vi "Set Tree Symbols.vi"(8 "error in":errorcluster, 10 "Tag":string, 11 "CtlRef":refnum<vi>) -> (0 "error out":errorcluster)   [LabVIEW 2015, in "J1939 Addon System Explorer.lvlib"]
uses:
  J1939 Addon System Explorer.lvlib
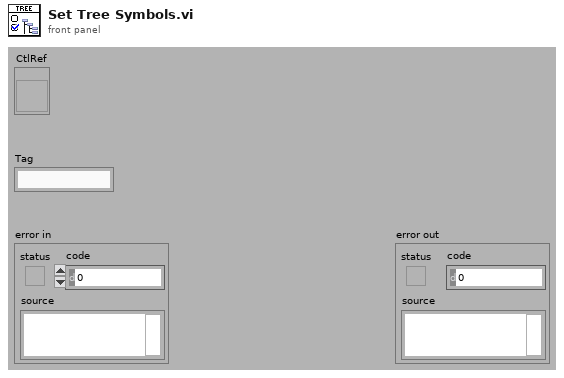
[diagram p1: front panel]
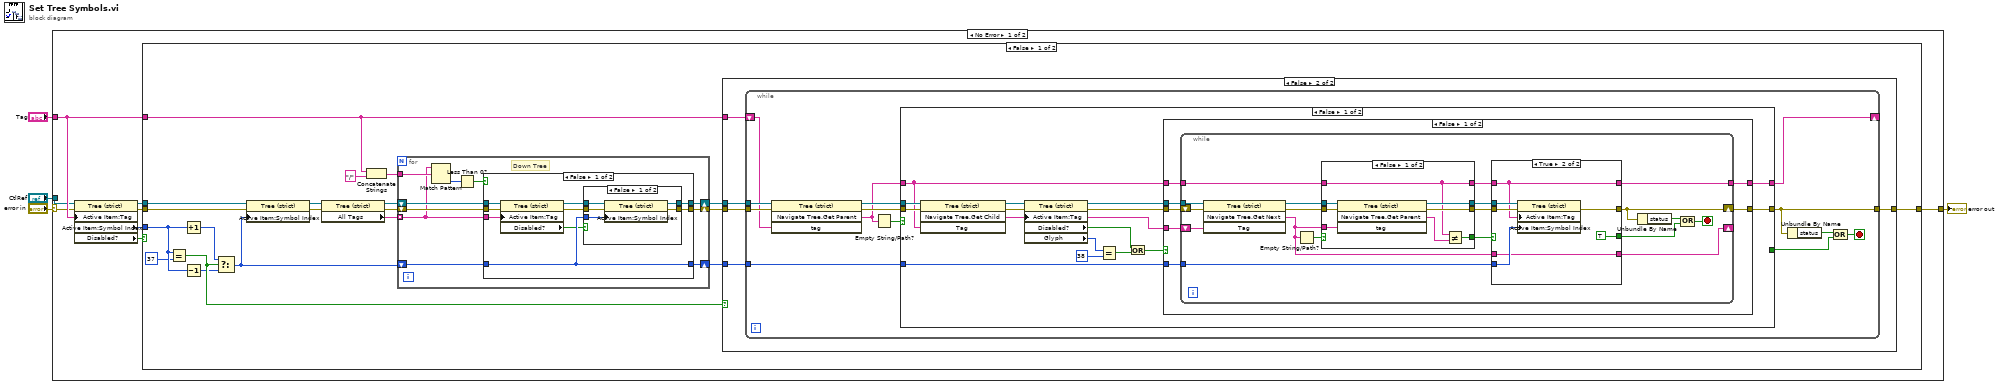
[diagram p0: block diagram]
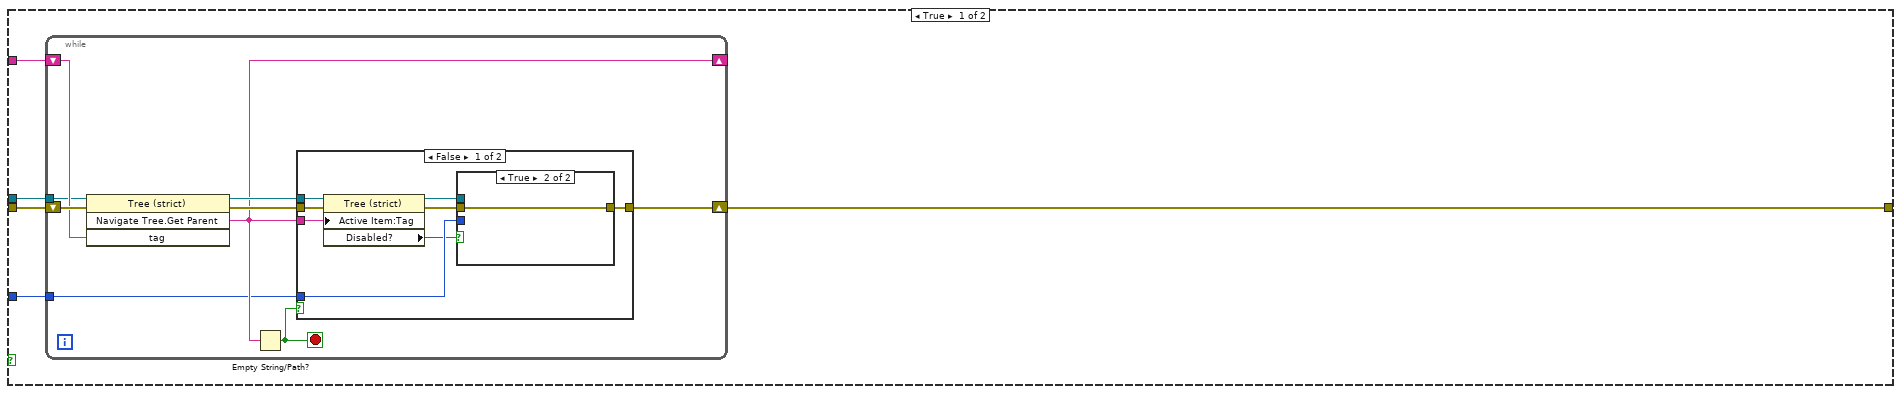
[diagram p2: hidden frame]
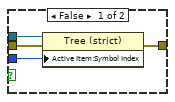
[diagram p3: hidden frame]
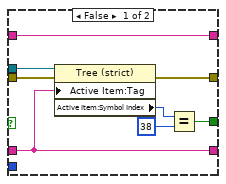
[diagram p6: hidden frame]
diagram:
  n1 = case shown="No Error" "error in" {
    selector: "error in" -> [w6 w183]
    tunnel: [w12 w183] -> w4
    tunnel: "Tag" -> [w11 _]
    tunnel: "CtlRef" -> [w10 _]
    frame No Error {
      n2 = property class="Tree (strict)"(reference=w10, error in=w6, "Active Item:Tag"=w11) -> (reference out=w8:refnum<vi>, error out=w9:errorcluster, "Active Item:Symbol Index"=w7:i32, "Disabled?"=w5:bool)
      n3 = case shown="False" w5 {
        tunnel: [w31 w182] -> w12
        tunnel: w11 -> [w29 _]
        tunnel: w9 -> [w18 w182]
        tunnel: w8 -> [w17 _]
        tunnel: w7 -> [w15 _]
        frame False {
          n4 = Equal?(x=w15, y=37 ("Active Item:Symbol Index")) -> (x = y?=w26:bool)
          n5 = Increment(x=w15) -> (x+1=w14:i32)
          n6 = Decrement(x=w15) -> (x-1=w16:i32)
          n7 = Select(t=w14, s=w26, f=w16) -> (s? t:f=w27:i32)
          n8 = property class="Tree (strict)"(reference=w17, error in=w18, "Active Item:Symbol Index"=w27) -> (reference out=w19:refnum<vi>, error out=w20:errorcluster)
          n9 = property class="Tree (strict)"(reference=w19, error in=w20) -> (reference out=w22:refnum<vi>, error out=w21:errorcluster, "All Tags"=w25:string[])
          n10 = Concatenate Strings(w29, "/" ("string")) -> (w24:string)
          n11 = for {
            tunnel: w24 -> [w162]
            tunnel: w25 -> [w155] mode=indexing
            shift-right: [w158] -> w28
            shift-left: w21 -> [w157]
            shift-right: [w154] -> w30
            shift-left: w22 -> [w156]
            shift-right: [w153] -> w32
            shift-left: w27 -> [w159]
            # "Down Tree"
            n12 = Match Pattern(string=w155, regular expression=w162) -> (offset past match=w161:i32)  [unwired: 1 in, 3 out]
            n13 = Less Than 0?(x=w161) -> (x < 0?=w160:bool)
            n14 = case shown="False" w160 {
              tunnel: w157 -> [w170 w181]
              tunnel: w156 -> [w171 w180]
              tunnel: w155 -> [w169 _]
              tunnel: w159 -> [w164 w179]
              tunnel: [w165 w181] -> w158
              tunnel: [w166 w180] -> w154
              tunnel: [w164 w179] -> w153
              frame False {
                n15 = property class="Tree (strict)"(reference=w171, error in=w170, "Active Item:Tag"=w169) -> (reference out=w167:refnum<vi>, error out=w168:errorcluster, "Disabled?"=w163:bool)
                n16 = case shown="False" w163 {
                  tunnel: w168 -> [w176 w177]
                  tunnel: w167 -> [w175 w178]
                  tunnel: [w174 w178] -> w166
                  tunnel: [w173 w177] -> w165
                  tunnel: w164 -> [w172 _]
                  frame False {
                    n17 = property class="Tree (strict)"(reference=w175, error in=w176, "Active Item:Symbol Index"=w172) -> (reference out=w174:refnum<vi>, error out=w173:errorcluster)
                  }
                  frame True {
                  }
                }
              }
              frame True {
              }
            }
          }
          n18 = case shown="False" w26 {
            tunnel: w28 -> [w37 w64]
            tunnel: w29 -> [w36 w62]
            tunnel: w30 -> [w35 w63]
            tunnel: [w34 w65] -> w31
            tunnel: w32 -> [w33 w61]
            frame True {
              n19 = while {
                tunnel: w35 -> [w44]
                shift-right: [w39] -> w34
                shift-left: w37 -> [w46]
                shift-right: [w41] -> _
                shift-left: w36 -> [w45]
                tunnel: w33 -> [w40]
                stop <- w38 stop-if-true
                n20 = invoke on="Invoke Node" class="Tree (strict)" method="Navigate Tree.Get Parent"(reference=w44, error in=w46, "tag"=w45) -> (reference out=w43:refnum<vi>, error out=w42:errorcluster, "Navigate Tree:Get Parent"=w41:string)  [unwired: 1 in, 1 out]
                n21 = Empty String/Path?(string/path=w41) -> (empty?=w38:bool)
                n22 = case shown="False" w38 {
                  tunnel: w42 -> [w53 w60]
                  tunnel: w43 -> [w54 _]
                  tunnel: w41 -> [w52 _]
                  tunnel: w40 -> [w48 _]
                  tunnel: [w49 w60] -> w39
                  frame False {
                    n23 = property class="Tree (strict)"(reference=w54, error in=w53, "Active Item:Tag"=w52) -> (reference out=w50:refnum<vi>, error out=w51:errorcluster, "Disabled?"=w47:bool)
                    n24 = case shown="True" w47 {
                      tunnel: w51 -> [w58 w59]
                      tunnel: w50 -> [w57 _]
                      tunnel: [w56 w59] -> w49
                      tunnel: w48 -> [w55 _]
                      frame False {
                        n25 = property class="Tree (strict)"(reference=w57, error in=w58, "Active Item:Symbol Index"=w55) -> (error out=w56:errorcluster)  [unwired: 1 out]
                      }
                      frame True {
                      }
                    }
                  }
                  frame True {
                  }
                }
              }
            }
            frame False {
              n26 = while {
                tunnel: [w69] -> w65
                tunnel: w64 -> [w78]
                tunnel: w63 -> [w77]
                shift-right: [w72] -> _
                shift-left: w62 -> [w71]
                tunnel: w61 -> [w70]
                stop <- w67 stop-if-true
                n27 = invoke on="Invoke Node" class="Tree (strict)" method="Navigate Tree.Get Parent"(reference=w77, error in=w78, "tag"=w71) -> (reference out=w75:refnum<vi>, error out=w76:errorcluster, "Navigate Tree:Get Parent"=w74:string)  [unwired: 1 in, 1 out]
                n28 = Empty String/Path?(string/path=w74) -> (empty?=w73:bool)
                n29 = case shown="False" w73 {
                  selector: w73 -> [_ w150]
                  tunnel: w70 -> [w94 _]
                  tunnel: [w93 w152] -> w69
                  tunnel: w76 -> [w92 w152]
                  tunnel: w75 -> [w91 _]
                  tunnel: w74 -> [w86 w151]
                  tunnel: [w84 w151] -> w72
                  tunnel: [_ w150] -> w66
                  frame False {
                    n30 = invoke on="Invoke Node" class="Tree (strict)" method="Navigate Tree.Get Child"(reference=w91, error in=w92, "Tag"=w86) -> (reference out=w90:refnum<vi>, error out=w88:errorcluster, "Navigate Tree:Get Child"=w79:string)  [unwired: 1 in, 1 out]
                    n31 = property class="Tree (strict)"(reference=w90, error in=w88, "Active Item:Tag"=w79) -> (reference out=w89:refnum<vi>, error out=w87:errorcluster, "Disabled?"=w82:bool, "Glyph"=w83:i32)
                    n32 = Equal?(x=w83, y=38 ("Active Item:Symbol Index")) -> (x = y?=w81:bool)
                    n33 = Or(x=w82, y=w81) -> (x .or. y?=w80:bool)
                    n34 = case shown="False" w80 {
                      tunnel: w94 -> [w101 _]
                      tunnel: [w100 w149] -> w93
                      tunnel: w89 -> [w99 _]
                      tunnel: w87 -> [w98 w149]
                      tunnel: w79 -> [w97 _]
                      tunnel: w86 -> [w96 w148]
                      tunnel: [w95 w148] -> w84
                      frame False {
                        n35 = while {
                          tunnel: w101 -> [w120]
                          tunnel: w99 -> [w117]
                          shift-right: [w107] -> w100
                          shift-left: w98 -> [w119]
                          shift-right: [w102] -> _
                          shift-left: w97 -> [w118]
                          tunnel: w96 -> [w108]
                          tunnel: [w103] -> w95
                          stop <- w105 stop-if-true
                          n36 = invoke on="Invoke Node" class="Tree (strict)" method="Navigate Tree.Get Next"(reference=w117, error in=w119, "Tag"=w118) -> (reference out=w116:refnum<vi>, error out=w114:errorcluster, "Navigate Tree:Get Next Item"=w109:string)  [unwired: 1 in, 1 out]
                          n37 = Empty String/Path?(string/path=w109) -> (empty?=w111:bool)
                          n38 = case shown="False" w111 {
                            selector: w111 -> [_ w132]
                            tunnel: w116 -> [w128 w130]
                            tunnel: [w127 w130] -> w115
                            tunnel: w114 -> [w126 w131]
                            tunnel: [w125 w131] -> w113
                            tunnel: [w123 w132] -> w112
                            tunnel: w108 -> [w121 w129]
                            tunnel: w109 -> [w122 _]
                            tunnel: [w121 w129] -> w110
                            frame False {
                              n39 = invoke on="Invoke Node" class="Tree (strict)" method="Navigate Tree.Get Parent"(reference=w128, error in=w126, "tag"=w122) -> (reference out=w127:refnum<vi>, error out=w125:errorcluster, "Navigate Tree:Get Parent"=w124:string)  [unwired: 1 in, 1 out]
                              n40 = Not Equal?(x=w121, y=w124) -> (x != y?=w123:bool)
                            }
                            frame True {
                            }
                          }
                          n41 = case shown="True" w112 {
                            tunnel: w120 -> [_ w143]
                            tunnel: w113 -> [w140 w145]
                            tunnel: [w135 w146] -> w107
                            tunnel: w115 -> [w139 w144]
                            tunnel: w109 -> [w133 w141]
                            tunnel: [w136 TRUE] -> w104
                            tunnel: w110 -> [w134 w142]
                            tunnel: [w134 w142] -> w103
                            tunnel: [w133 w141] -> w102
                            frame False {
                              n42 = property class="Tree (strict)"(reference=w139, error in=w140, "Active Item:Tag"=w133) -> (error out=w135:errorcluster, "Active Item:Symbol Index"=w137:i32)  [unwired: 1 out]
                              n43 = Equal?(x=w137, y=38 ("Active Item:Symbol Index")) -> (x = y?=w136:bool)
                            }
                            frame True {
                              n44 = property class="Tree (strict)"(reference=w144, error in=w145, "Active Item:Tag"=w142, "Active Item:Symbol Index"=w143) -> (error out=w146:errorcluster)  [unwired: 1 out]
                            }
                          }
                          n45 = Unbundle By Name(w107) -> ("status"=w106:bool)
                          n46 = Compound Arithmetic op=OR(w106, w104) -> (w105:bool)
                        }
                      }
                      frame True {
                      }
                    }
                  }
                  frame True {
                  }
                }
                n47 = Unbundle By Name(w69) -> ("status"=w68:bool)
                n48 = Compound Arithmetic op=OR(w68, w66) -> (w67:bool)
              }
            }
          }
        }
        frame True {
        }
      }
    }
    frame Error {
    }
  }
  "error out" <- w4
